vi "PicoScope2000aGetBlock.vi"(0 "error in":errorcluster, 2 "handle in":i16, 3 "Acquisition Settings":T4, 5 "enabled array":i16[](array[numeric]), 8 "Buffer and Transfer Settings":T1 {"Down-Sample Mode" items=["None", "Aggregate", "Decimate", "Average"]; "Down Sample Ratio" step=1; "Samples" format="%_6p"}) -> (1 "noOfSamples":u64, 4 "overflow":i16, 6 "error out":errorcluster, 7 "handle out":i16, 9 "Buffers (Max or non-aggregated)":T2, 10 "Min Buffers":T3)   [LabVIEW 2009]
doc: "This VI collects a block of data from the oscilloscope. This can be called in a loop in order to continually collect blocks of data. The oscilloscope should first be set up by using PicoScope3000aSettings.vi. The VI outputs data arrays in two clusters (max and min). If not using aggregation, 'Min Buffers' is not used."
uses:
  ps2000a.dll
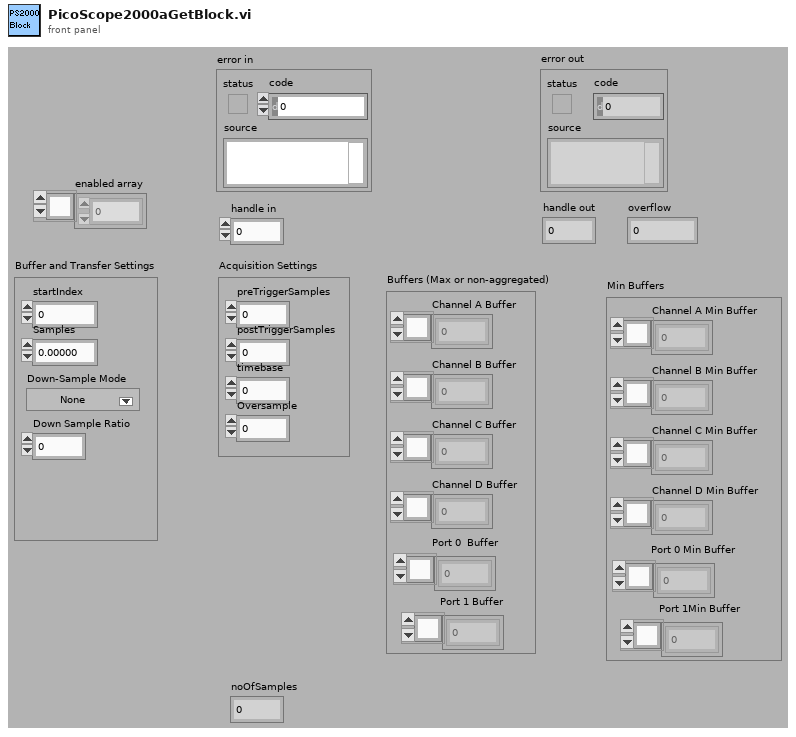
[diagram p1: front panel]
types:
  T1 = cluster{"startIndex":u64, "Samples":u64, "Down Sample Ratio":u64, "Down-Sample Mode":u32}
  T2 = cluster{"Channel D Buffer":i16[], "Channel C Buffer":i16[], "Channel B Buffer":i16[], "Channel A Buffer":i16[], "Port 0  Buffer ":i16[], "Port 1 Buffer ":i16[]}
  T3 = cluster{"Channel A Min Buffer":i16[], "Channel B Min Buffer":i16[], "Channel C Min Buffer":i16[], "Channel D Min Buffer":i16[], "Port 0 Min Buffer ":i16[], "Port 1Min Buffer ":i16[]}
  T4 = cluster{"preTriggerSamples":u32, "postTriggerSamples":u32, "timebase":u32, "Oversample":i16}
  T5 = cluster{"Channel A Min Buffer":i16[], "Channel B Min Buffer":i16[], "Channel C Min Buffer":i16[], "Channel D Min Buffer":i16[], "Port 0 Min Buffer":i32[], "Port 1 Min Buffer":i32[]}
  T6 = cluster{"Channel D Buffer":i16[], "Channel C Buffer":i16[], "Channel B Buffer":i16[], "Channel A Buffer":i16[], "Port 0 Max Buffer":i32[], "Port 1 Max Buffer":i32[]}
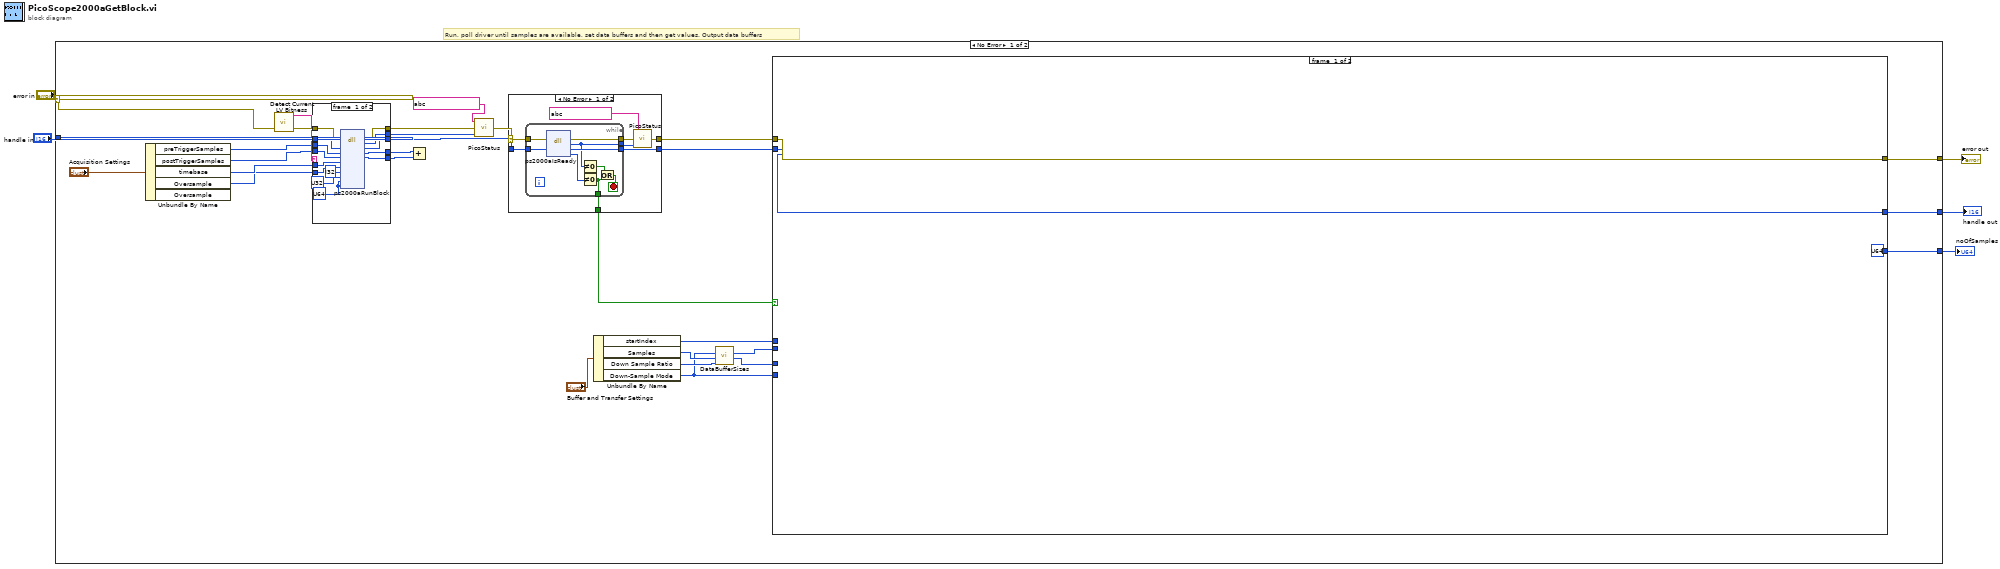
[diagram p0: block diagram]
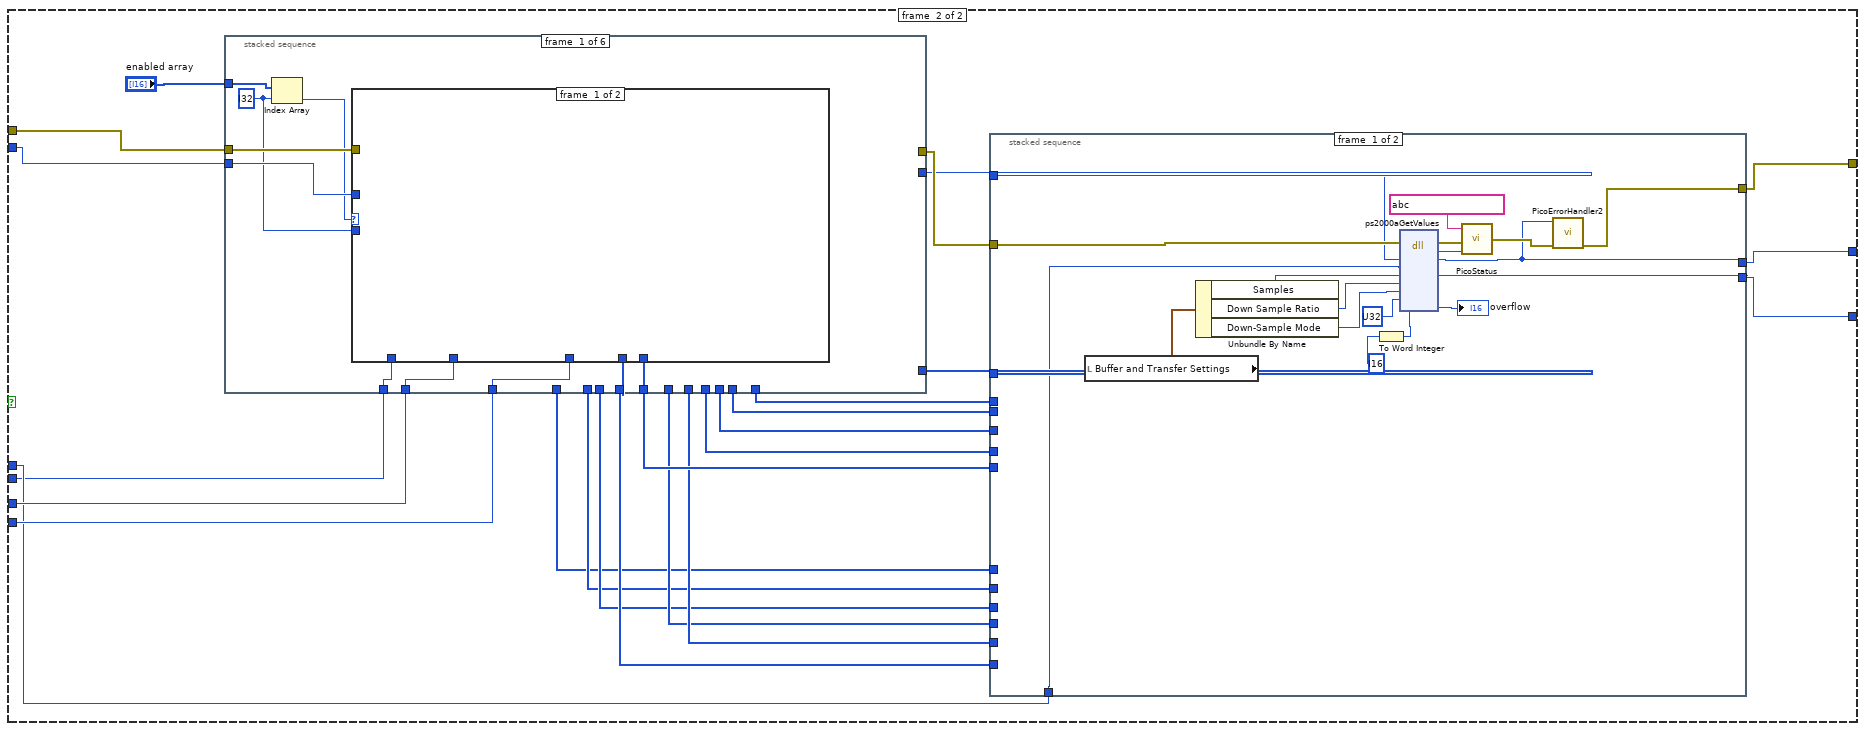
[diagram p2: hidden frame]
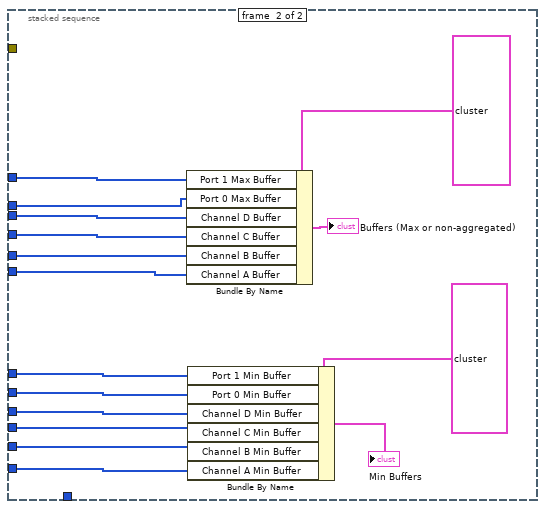
[diagram p3: hidden frame]
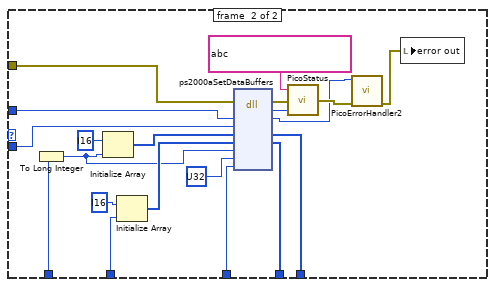
[diagram p4: hidden frame]
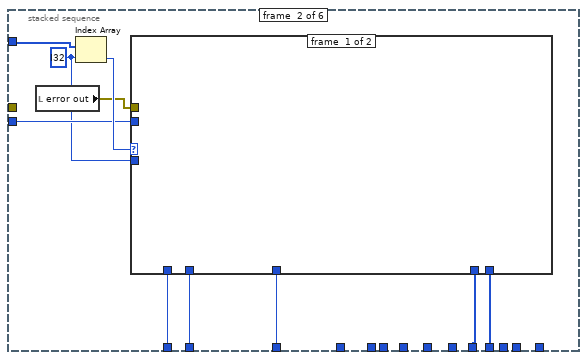
[diagram p5: hidden frame]
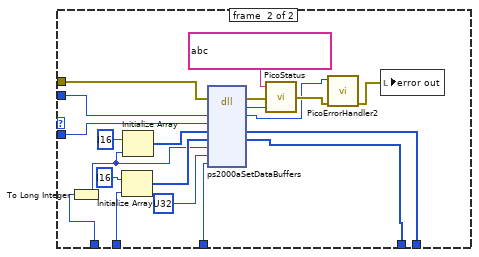
[diagram p6: hidden frame]
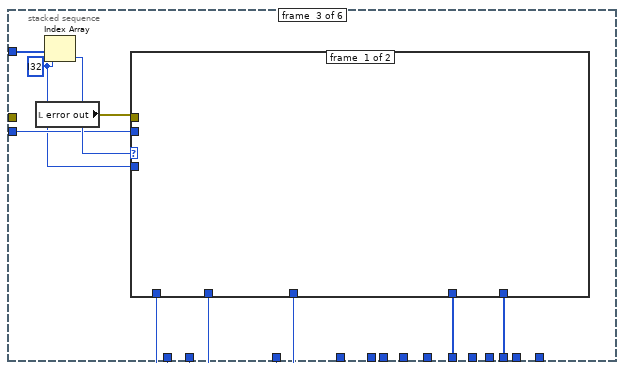
[diagram p7: hidden frame]
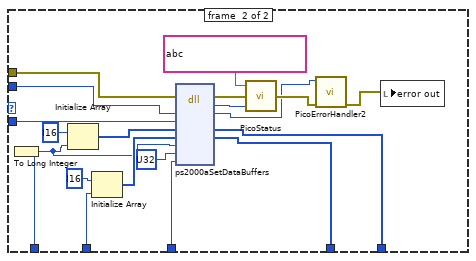
[diagram p8: hidden frame]
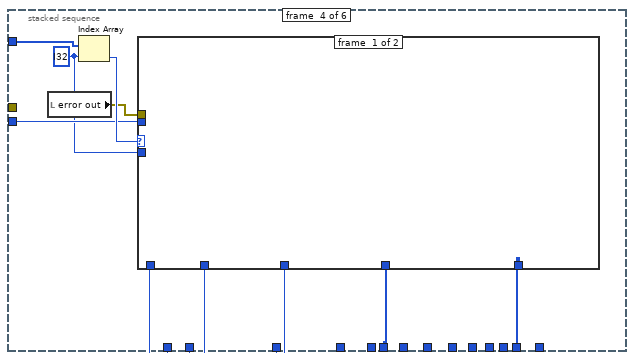
[diagram p9: hidden frame]
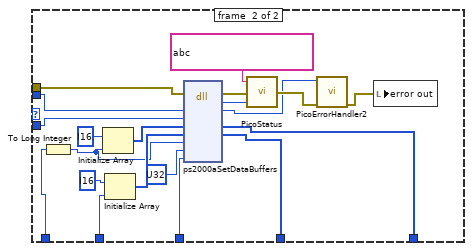
[diagram p10: hidden frame]
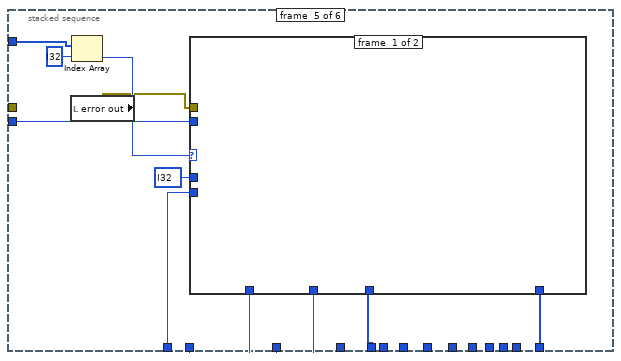
[diagram p11: hidden frame]
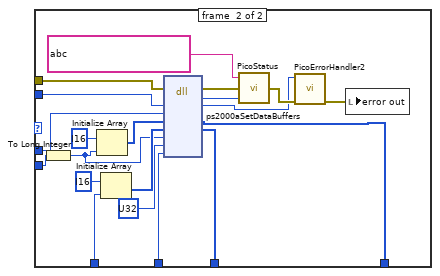
[diagram p12: hidden frame]
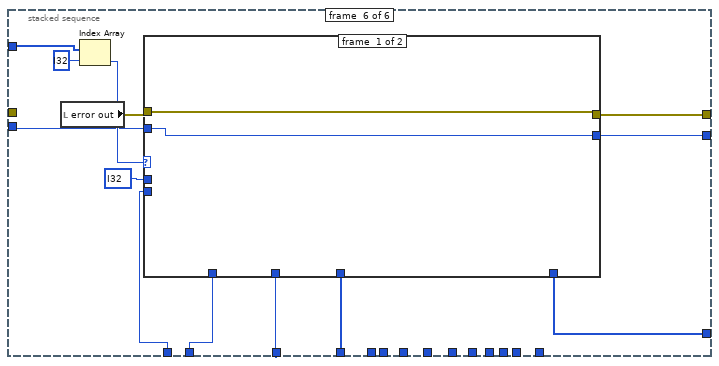
[diagram p13: hidden frame]
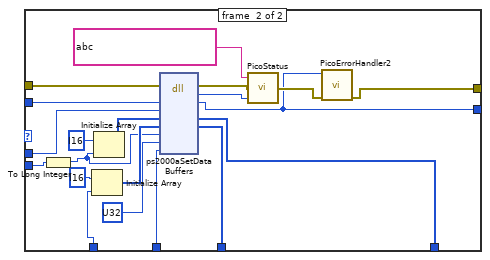
[diagram p14: hidden frame]
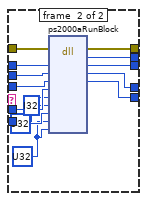
[diagram p15: hidden frame]
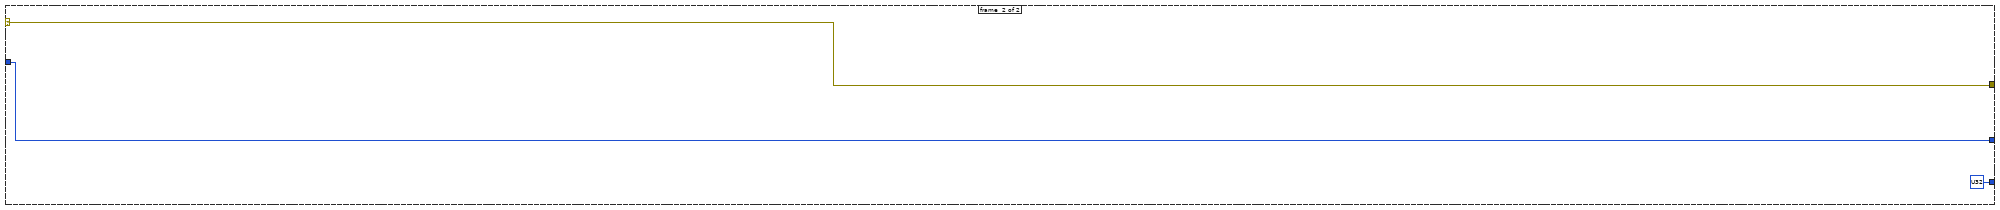
[diagram p17: hidden frame]
diagram:
  # "Run, poll driver until samples are available, set data buffers and then get values. Output data buffers"
  n1 = case shown="No Error" "error in" {
    selector: "error in" -> [w25 w330]
    tunnel: [w9 w330] -> w1
    tunnel: "handle in" -> [w21 w329]
    tunnel: [w7 u32 ? ("noOfSamples")] -> w3
    tunnel: [w6 w329] -> w2
    frame #0 {
      n2 = Unbundle By Name("Acquisition Settings") -> ("preTriggerSamples"=w20:u32, "postTriggerSamples"=w19:u32, "timebase"=w18:u32, "Oversample"=w17:i16)  [unwired: 1 out]
      n3 = call "Detect Current LV Bitness.vi"() -> ("bitness"=w24:string)  [unwired: 11 in]
      n4 = case shown="\"32\", Default" w24 {
        tunnel: [w291 w308] -> w33
        tunnel: [w292 w307] -> w29
        tunnel: [w293 w306] -> w28
        tunnel: w25 -> [w294 w305]
        tunnel: [w290 w304] -> w23
        tunnel: [w289 w303] -> w22
        tunnel: w21 -> [w287 w302]
        tunnel: w20 -> [w286 w301]
        tunnel: w19 -> [w285 w300]
        tunnel: w18 -> [w284 w299]
        tunnel: w17 -> [w283 w298]
        frame #0 {
          w288 = u64 ? ("pParameter")
          n5 = dll-call lib="ps2000a.dll" fn="ps2000aRunBlock" ("ps3000.dll:_ps3000_open_unit@0")(error in=w294, "handle"=w287, "preTriggerSamples"=w286, "postTriggerSamples"=w285, "timebase"=w284, "oversample"=w283, "timeindisposed"=i32 ?, "segmentIndex"=u32 ?, "lpReady"=w288, "pParameter"=w288) -> (error out=w293:errorcluster, "PICO_STATUS"=w292:i32, "handle"=w291:i16, "preTriggerSamples"=w290:u32, "postTriggerSamples"=w289:u32)  [unwired: 8 in, 1 out]
        }
        frame #1 {
          w295 = u32 ? ("lpReady")
          n6 = dll-call lib="ps2000a.dll" fn="ps2000aRunBlock" ("ps3000.dll:_ps3000_open_unit@0")(error in=w305, "handle"=w302, "preTriggerSamples"=w301, "postTriggerSamples"=w300, "timebase"=w299, "oversample"=w298, "timeindisposed"=i32 ?, "segmentIndex"=u32 ?, "lpReady"=w295, "pParameter"=w295) -> (error out=w306:errorcluster, "PICO_STATUS"=w307:u32, "handle"=w308:i16, "preTriggerSamples"=w304:u32, "postTriggerSamples"=w303:u32)  [unwired: 8 in, 1 out]
        }
      }
      n7 = Add(x=w23, y=w22) -> ()  [unwired: 1 out]
      n8 = call "PicoStatus.vi"("PICO STATUS"=w29, "error in"=w28, "source"=string ?) -> ("error out"=w27:errorcluster)
      n9 = case shown="No Error" w27 {
        selector: w27 -> [w314 w326]
        tunnel: w33 -> [w316 w327]
        tunnel: [w315 w327] -> w32
        tunnel: [w313 w326] -> w31
        tunnel: [w309 _] -> w13
        frame #0 {
          n10 = while {
            tunnel: [w325] -> w315
            tunnel: w316 -> [w324]
            tunnel: [w320] -> w311
            tunnel: w314 -> [w319]
            tunnel: [w318] -> w312
            tunnel: [w317] -> w309
            stop <- w323 stop-if-true
            n11 = dll-call lib="ps2000a.dll" fn="ps2000aIsReady" ("ps3000.dll:_ps3000_open_unit@0")(error in=w319, "handle"=w324) -> (error out=w318:errorcluster, "status"=w320:u32, "handle"=w325:i16, "ready"=w321:i16)  [unwired: 3 in, 1 out]
            n12 = Not Equal To 0?(x=w320) -> (x != 0?=w322:bool)
            n13 = Not Equal To 0?(x=w321) -> (x != 0?=w317:bool)
            n14 = Or(x=w322, y=w317) -> (x .or. y?=w323:bool)
          }
          n15 = call "PicoStatus.vi"("PICO STATUS"=w311, "error in"=w312, "source"=string ?) -> ("error out"=w313:errorcluster)
        }
        frame #1 {
        }
      }
      n16 = Unbundle By Name("Buffer and Transfer Settings") -> ("startIndex"=w8:u64, "Samples"=w15:u64, "Down Sample Ratio"=w14:u64, "Down-Sample Mode"=w12:u32)
      n17 = call "DataBufferSizes.vi"("Down Sample Ratio"=w14, "Number of Samples"=w15, "Down-Sample Mode"=w12) -> ("min Buffer Size"=w10:i32, "Max Buffer Size"=w11:i32)  [unwired: 7 in]
      n18 = case shown="True" w13 {
        tunnel: w32 -> [w35 w60]
        tunnel: w31 -> [w36 w59]
        tunnel: w12 -> [_ w57]
        tunnel: w11 -> [_ w37]
        tunnel: w10 -> [_ w56]
        tunnel: [w36 w55] -> w9
        tunnel: w8 -> [_ w38]
        tunnel: [u64 ? ("noOfSamples") w40] -> w7
        tunnel: [w35 w39] -> w6
        frame #0 {
        }
        frame #1 {
          n19 = stacked-sequence {
            tunnel: w60 -> [w104 w132 w162 w192 w223 w255]
            tunnel: w59 -> [w103 _ _ _ _ _]
            tunnel: "enabled array" -> [w102 w134 w164 w194 w225 w258]
            tunnel: w57 -> [w99 w130 w160 w188 w220 w253]
            tunnel: w37 -> [w98 w129 w159 w190 w222 w254]
            tunnel: w56 -> [w97 w128 w158 w189 w221 w252]
            tunnel: [w96 _ _ _ _ _] -> w54
            tunnel: [w95 _ _ _ _ _] -> w53
            tunnel: [_ w126 _ _ _ _] -> w52
            tunnel: [_ w125 _ _ _ _] -> w51
            tunnel: [_ _ w156 _ _ _] -> w50
            tunnel: [_ _ w155 _ _ _] -> w49
            tunnel: [_ _ _ w186 _ _] -> w48
            tunnel: [_ _ _ w185 _ _] -> w47
            tunnel: [_ _ _ _ w218 _] -> w46
            tunnel: [_ _ _ _ w217 _] -> w45
            tunnel: [_ _ _ _ _ w250] -> w44
            tunnel: [_ _ _ _ _ w249] -> w43
            tunnel: [_ _ _ _ _ w248] -> w42
            tunnel: [_ _ _ _ _ w247] -> w41
            frame #0 {
              w100 = i32 ? ("dimension size")
              n20 = Index Array(array=w102, index=w100) -> (element=w101:i16)
              n21 = case shown="1" w101 {
                tunnel: w104 -> [_ w124]
                tunnel: w103 -> [_ w121]
                tunnel: w100 -> [_ w115]
                tunnel: w99 -> [_ w114]
                tunnel: w98 -> [_ w113]
                tunnel: w97 -> [_ w112]
                tunnel: [_ w110] -> w96
                tunnel: [_ w109] -> w95
                frame #0 {
                }
                frame #1 {
                  n22 = To Long Integer(number=w113) -> (32bit integer=w105:i32)
                  n23 = Initialize Array(i16 ? ("element"), w105) -> (w123:i16[])
                  n24 = Initialize Array(i16 ? ("element"), w112) -> (w116:i16[])
                  n25 = dll-call lib="ps2000a.dll" fn="ps2000aSetDataBuffers" ("ps3000.dll:_ps3000_open_unit@0")(error in=w121, "handle"=w124, "channel"=w115, "bufferMax"=w123, "bufferMin"=w116, "bufferLth"=w105, "segmentIndex"=u32 ?, "mode"=w114) -> (error out=w119:errorcluster, "PICO_STATUS"=w120:u32, "handle"=w107:i16, "bufferMax"=w110:i16[], "bufferMin"=w109:i16[])  [unwired: 6 in, 1 out]
                  n26 = call "PicoStatus.vi"("PICO STATUS"=w120, "error in"=w119, "source"=string ?) -> ("error out"=w108:errorcluster)
                  n27 = call "PicoErrorHandler2.vi"("error in (no error)"=w108, "handle In"=w107) -> ("error out"=w106:errorcluster)  [unwired: 9 in]
                  n28 = local write "error out"(w106) -> ()
                }
              }
            }
            frame #1 {
              w131 = i32 ? ("dimension size")
              n29 = local read "error out"() -> (w127:errorcluster)
              n30 = Index Array(array=w134, index=w131) -> (element=w133:i16)
              n31 = case shown="1" w133 {
                tunnel: w127 -> [_ w147]
                tunnel: w132 -> [_ w146]
                tunnel: w131 -> [_ w145]
                tunnel: w130 -> [_ w144]
                tunnel: w129 -> [_ w142]
                tunnel: w128 -> [_ w143]
                tunnel: [_ w137] -> w126
                tunnel: [_ w136] -> w125
                frame #0 {
                }
                frame #1 {
                  n32 = To Long Integer(number=w142) -> (32bit integer=w135:i32)
                  n33 = Initialize Array(i16 ? ("element"), w143) -> (w148:i16[])
                  n34 = Initialize Array(i16 ? ("element"), w135) -> (w154:i16[])
                  n35 = dll-call lib="ps2000a.dll" fn="ps2000aSetDataBuffers" ("ps3000.dll:_ps3000_open_unit@0")(error in=w147, "handle"=w146, "channel"=w145, "bufferMax"=w154, "bufferMin"=w148, "bufferLth"=w135, "segmentIndex"=u32 ?, "mode"=w144) -> (error out=w151:errorcluster, "PICO_STATUS"=w152:i32, "handle"=w139:i16, "bufferMax"=w137:i16[], "bufferMin"=w136:i16[])  [unwired: 6 in, 1 out]
                  n36 = call "PicoStatus.vi"("PICO STATUS"=w152, "error in"=w151, "source"=string ?) -> ("error out"=w140:errorcluster)
                  n37 = call "PicoErrorHandler2.vi"("error in (no error)"=w140, "handle In"=w139) -> ("error out"=w138:errorcluster)  [unwired: 9 in]
                  n38 = local write "error out"(w138) -> ()
                }
              }
            }
            frame #2 {
              w161 = i32 ? ("dimension size")
              n39 = local read "error out"() -> (w157:errorcluster)
              n40 = Index Array(array=w164, index=w161) -> (element=w163:i16)
              n41 = case shown="1" w163 {
                tunnel: w157 -> [_ w177]
                tunnel: w162 -> [_ w176]
                tunnel: w161 -> [_ w175]
                tunnel: w160 -> [_ w174]
                tunnel: w159 -> [_ w173]
                tunnel: w158 -> [_ w172]
                tunnel: [_ w168] -> w156
                tunnel: [_ w167] -> w155
                frame #0 {
                }
                frame #1 {
                  n42 = To Long Integer(number=w173) -> (32bit integer=w165:i32)
                  n43 = Initialize Array(i16 ? ("element"), w165) -> (w184:i16[])
                  n44 = Initialize Array(i16 ? ("element"), w172) -> (w178:i16[])
                  n45 = dll-call lib="ps2000a.dll" fn="ps2000aSetDataBuffers" ("ps3000.dll:_ps3000_open_unit@0")(error in=w177, "handle"=w176, "channel"=w175, "bufferMax"=w184, "bufferMin"=w178, "bufferLth"=w165, "segmentIndex"=u32 ?, "mode"=w174) -> (error out=w181:errorcluster, "PICO_STATUS"=w182:i32, "handle"=w170:i16, "bufferMax"=w168:i16[], "bufferMin"=w167:i16[])  [unwired: 6 in, 1 out]
                  n46 = call "PicoStatus.vi"("PICO STATUS"=w182, "error in"=w181, "source"=string ?) -> ("error out"=w171:errorcluster)
                  n47 = call "PicoErrorHandler2.vi"("error in (no error)"=w171, "handle In"=w170) -> ("error out"=w169:errorcluster)  [unwired: 9 in]
                  n48 = local write "error out"(w169) -> ()
                }
              }
            }
            frame #3 {
              w191 = i32 ? ("dimension size")
              n49 = local read "error out"() -> (w187:errorcluster)
              n50 = Index Array(array=w194, index=w191) -> (element=w193:i16)
              n51 = case shown="1" w193 {
                tunnel: w192 -> [_ w207]
                tunnel: w191 -> [_ w206]
                tunnel: w190 -> [_ w205]
                tunnel: w189 -> [_ w204]
                tunnel: w188 -> [_ w203]
                tunnel: w187 -> [_ w201]
                tunnel: [_ w197] -> w186
                tunnel: [_ w196] -> w185
                frame #0 {
                }
                frame #1 {
                  n52 = To Long Integer(number=w205) -> (32bit integer=w195:i32)
                  n53 = Initialize Array(i16 ? ("element"), w195) -> (w214:i16[])
                  n54 = Initialize Array(i16 ? ("element"), w204) -> (w208:i16[])
                  n55 = dll-call lib="ps2000a.dll" fn="ps2000aSetDataBuffers" ("ps3000.dll:_ps3000_open_unit@0")(error in=w201, "handle"=w207, "channel"=w206, "bufferMax"=w214, "bufferMin"=w208, "bufferLth"=w195, "segmentIndex"=u32 ?, "mode"=w203) -> (error out=w211:errorcluster, "PICO_STATUS"=w212:i32, "handle"=w198:i16, "bufferMax"=w197:i16[], "bufferMin"=w196:i16[])  [unwired: 6 in, 1 out]
                  n56 = call "PicoStatus.vi"("PICO STATUS"=w212, "error in"=w211, "source"=string ?) -> ("error out"=w199:errorcluster)
                  n57 = call "PicoErrorHandler2.vi"("error in (no error)"=w199, "handle In"=w198) -> ("error out"=w200:errorcluster)  [unwired: 9 in]
                  n58 = local write "error out"(w200) -> ()
                }
              }
            }
            frame #4 {
              n59 = local read "error out"() -> (w219:errorcluster)
              n60 = Index Array(array=w225, index=i32 ? ("dimension size")) -> (element=w224:i16)
              n61 = case shown="1" w224 {
                tunnel: i32 ? ("dimension size") -> [_ w245]
                tunnel: w219 -> [_ w242]
                tunnel: w223 -> [_ w241]
                tunnel: w222 -> [_ w237]
                tunnel: w221 -> [_ w236]
                tunnel: w220 -> [_ w233]
                tunnel: [_ w228] -> w218
                tunnel: [_ w227] -> w217
                frame #0 {
                }
                frame #1 {
                  n62 = To Long Integer(number=w237) -> (32bit integer=w226:i32)
                  n63 = Initialize Array(i16 ? ("element"), w226) -> (w238:i16[])
                  n64 = Initialize Array(i16 ? ("element"), w236) -> (w235:i16[])
                  n65 = dll-call lib="ps2000a.dll" fn="ps2000aSetDataBuffers" ("ps3000.dll:_ps3000_open_unit@0")(error in=w242, "handle"=w241, "channel"=w245, "bufferMax"=w238, "bufferMin"=w235, "bufferLth"=w226, "segmentIndex"=u32 ?, "mode"=w233) -> (error out=w244:errorcluster, "PICO_STATUS"=w230:u32, "handle"=w229:i16, "bufferMax"=w228:i16[], "bufferMin"=w227:i16[])  [unwired: 6 in, 1 out]
                  n66 = call "PicoStatus.vi"("PICO STATUS"=w230, "error in"=w244, "source"=string ?) -> ("error out"=w232:errorcluster)
                  n67 = call "PicoErrorHandler2.vi"("error in (no error)"=w232, "handle In"=w229) -> ("error out"=w231:errorcluster)  [unwired: 9 in]
                  n68 = local write "error out"(w231) -> ()
                }
              }
            }
            frame #5 {
              n69 = local read "error out"() -> (w251:errorcluster)
              n70 = Index Array(array=w258, index=i32 ? ("dimension size")) -> (element=w257:i16)
              n71 = case shown="1" w257 {
                tunnel: i32 ? -> [_ w277]
                tunnel: w251 -> [w260 w274]
                tunnel: w255 -> [w259 w273]
                tunnel: w254 -> [_ w271]
                tunnel: w253 -> [_ w269]
                tunnel: w252 -> [_ w268]
                tunnel: [_ w265] -> w250
                tunnel: [_ w264] -> w249
                tunnel: [w260 w263] -> w248
                tunnel: [w259 w262] -> w247
                frame #0 {
                }
                frame #1 {
                  n72 = To Long Integer(number=w271) -> (32bit integer=w261:i32)
                  n73 = Initialize Array(i16 ? ("element"), w268) -> (w270:i16[])
                  n74 = Initialize Array(i16 ? ("element"), w261) -> (w272:i16[])
                  n75 = dll-call lib="ps2000a.dll" fn="ps2000aSetDataBuffers" ("ps3000.dll:_ps3000_open_unit@0")(error in=w274, "handle"=w273, "channel"=w277, "bufferMax"=w272, "bufferMin"=w270, "bufferLth"=w261, "segmentIndex"=u32 ?, "mode"=w269) -> (error out=w280:errorcluster, "PICO_STATUS"=w278:u32, "handle"=w262:i16, "bufferMax"=w265:i16[], "bufferMin"=w264:i16[])  [unwired: 6 in, 1 out]
                  n76 = call "PicoStatus.vi"("PICO STATUS"=w278, "error in"=w280, "source"=string ?) -> ("error out"=w266:errorcluster)
                  n77 = call "PicoErrorHandler2.vi"("error in (no error)"=w266, "handle In"=w262) -> ("error out"=w263:errorcluster)  [unwired: 9 in]
                }
              }
            }
          }
          n78 = stacked-sequence {
            tunnel: [w69 _] -> w55
            tunnel: w54 -> [_ w90]
            tunnel: w53 -> [_ w89]
            tunnel: w52 -> [_ w88]
            tunnel: w51 -> [_ w87]
            tunnel: w50 -> [_ w86]
            tunnel: w49 -> [_ w85]
            tunnel: w48 -> [_ w84]
            tunnel: w47 -> [_ w83]
            tunnel: w46 -> [_ w82]
            tunnel: w45 -> [_ w81]
            tunnel: w44 -> [_ w80]
            tunnel: w43 -> [_ w79]
            tunnel: w42 -> [w74 _]
            tunnel: w41 -> [w73 _]
            tunnel: [w70 _] -> w39
            tunnel: [w72 _] -> w40
            tunnel: w38 -> [w63 _]
            frame #0 {
              n79 = local read "Buffer and Transfer Settings"() -> (w67:T1)
              n80 = Unbundle By Name(w67) -> ("Samples"=w66:u64, "Down Sample Ratio"=w65:u64, "Down-Sample Mode"=w64:u32)
              n81 = To Word Integer(number=i16 ? ("overflow")) -> (16bit integer=w61:i16)
              n82 = dll-call lib="ps2000a.dll" fn="ps2000aGetValues" ("ps3000.dll:_ps3000_open_unit@0")(error in=w74, "handle"=w73, "startIndex"=w63, "noOfSamples"=w66, "downSampleRatio"=w65, "downSampleRatioMode"=w64, "segmentIndex"=u32 ?, "overflow"=w61) -> (error out=w76:errorcluster, "PICO_STATUS"=w77:u32, "handle"=w70:i16, "noOfSamples"=w72:u64, "overflow"=→"overflow":i16)  [unwired: 6 in, 1 out]
              n83 = call "PicoStatus.vi"("PICO STATUS"=w77, "error in"=w76, "source"=string ?) -> ("error out"=w71:errorcluster)
              n84 = call "PicoErrorHandler2.vi"("error in (no error)"=w71, "handle In"=w70) -> ("error out"=w69:errorcluster)  [unwired: 9 in]
            }
            frame #1 {
              n85 = Bundle By Name(cluster=T6 ? ("Buffers (Max or non-aggregated)"), "Port 1 Max Buffer"=w80, "Port 0 Max Buffer"=w82, "Channel D Buffer"=w84, "Channel C Buffer"=w86, "Channel B Buffer"=w88, "Channel A Buffer"=w90) -> (→"Buffers (Max or non-aggregated)":T6)
              n86 = Bundle By Name(cluster=T5 ? ("Min Buffers"), "Port 1 Min Buffer"=w79, "Port 0 Min Buffer"=w81, "Channel D Min Buffer"=w83, "Channel C Min Buffer"=w85, "Channel B Min Buffer"=w87, "Channel A Min Buffer"=w89) -> (→"Min Buffers":T5)
            }
          }
        }
      }
    }
    frame #1 {
    }
  }
  "error out" <- w1
  "handle out" <- w2
  "noOfSamples" <- w3
